vi "Test_Press_Hist.vi"() -> ()   [LabVIEW 2016]
uses:
  <userlib>/Fluigent/Fluigent MFCS/FluigentMFCS_Full.llb/MFCS_EZ Detect.vi
  <userlib>/Fluigent/Fluigent MFCS/FluigentMFCS_Full.llb/MFCS_EZ Initialization.vi
  <userlib>/Fluigent/Fluigent MFCS/FluigentMFCS_Full.llb/MFCS_EZ Read All Channels Pressure.vi
  <vilib>/imath/engines/lvmath2/RunTimeEngine/BuiltInFunctions/sets_unique/NIMS_sets_unique(GV).vi
  <instcachedir>/0/NIMS_sets_unique(GV)_BC60CBD939E647F382369330BF9EA64D.lvgen/NIMS_sets_unique(GV)_BC60CBD939E647F382369330BF9EA64D_001.vi
  <vilib>/imath/engines/lvmath2/RunTimeEngine/BuiltInFunctions/size/NIMS_I32Row=size(GRow).vi
  <instcachedir>/0/NIMS_I32Row=size(GRow)_E5C05C6B13124B29B774CC4F993D3C59.lvgen/NIMS_I32Row=size(GRow)_E5C05C6B13124B29B774CC4F993D3C59_000.vi
  <vilib>/imath/engines/lvmath2/RunTimeEngine/BuiltInFunctions/zeros/NIMS_M=zeros(I32V).vi
  <vilib>/imathl/engines/lvmath/Functions/Error Handling/Create Error.vi
  <vilib>/imath/engines/lvmath2/RunTimeEngine/BuiltInFunctions/length/NIMS_length(GV).vi
  <instcachedir>/0/NIMS_length(GV)_08A3D13377FD4E4B96F5795FBF3698FA.lvgen/NIMS_length(GV)_08A3D13377FD4E4B96F5795FBF3698FA_000.vi
  <vilib>/imath/engines/lvmath2/RunTimeEngine/RangeToken/NIMS_Range_R2 - Integer.vi
  <instcachedir>/0/NIMS_Range_R2 - Integer_416A044C4F024DBE8E97DA138CB3186F.lvgen/NIMS_Range_R2 - Integer_416A044C4F024DBE8E97DA138CB3186F_000.vi
  <vilib>/imath/engines/lvmath2/RunTimeEngine/CommandStatement/MC_CommandStatement_break.vi
  <vilib>/imath/engines/lvmath2/RunTimeEngine/IndexRead/NIMS V(S).vi
  <instcachedir>/0/NIMS V(S)_0488751826AF41519A22953C041130DC.lvgen/NIMS V(S)_0488751826AF41519A22953C041130DC_000.vi
  <vilib>/imath/engines/lvmath2/RunTimeEngine/BuiltInFunctions/findnz/NIMS_[1o]_findnz(GRowV).vi
  <instcachedir>/0/NIMS_[1o]_findnz(GRowV)_656056C849EF4762B1F0843BDDDEF2FF.lvgen/NIMS_[1o]_findnz(GRowV)_656056C849EF4762B1F0843BDDDEF2FF_000.vi
  <instcachedir>/0/NIMS_length(GV)_08A3D13377FD4E4B96F5795FBF3698FA.lvgen/NIMS_length(GV)_08A3D13377FD4E4B96F5795FBF3698FA_002.vi
  <vilib>/imath/engines/lvmath2/RunTimeEngine/IndexReplace/NIMS M(S)=S.vi
  <instcachedir>/0/NIMS M(S)=S_9328EF344EC9443A8B5E4239F1A18A91.lvgen/NIMS M(S)=S_9328EF344EC9443A8B5E4239F1A18A91_000.vi
  <vilib>/imath/engines/lvmath2/RunTimeEngine/ErrorHandling/NIMS_Create Error From Enums.vi
  <vilib>/imath/engines/lvmath2/RunTimeEngine/BuiltInFunctions/difference/NIMS_difference(GV,I32).vi
  <instcachedir>/0/NIMS_difference(GV,I32)_DC7351DCBCF840A8AE147F50EC2CE86E.lvgen/NIMS_difference(GV,I32)_DC7351DCBCF840A8AE147F50EC2CE86E_000.vi
  <vilib>/imath/engines/lvmath2/RunTimeEngine/NodeEndStatement/NIMS_NodeEndStatement_Get Vector.vi
  <instcachedir>/0/NIMS_NodeEndStatement_Get Vector_6D35898B950C4E42AD3C631ACA708625.lvgen/NIMS_NodeEndStatement_Get Vector_6D35898B950C4E42AD3C631ACA708625_000.vi
  <vilib>/imath/engines/lvmath/Functions/Error Handling/MergeErrorsWrapper.vi
  <vilib>/imath/engines/lvmath2/RunTimeEngine/NodeEndStatement/NIMS_NodeEndStatement_Output.vi
  <instcachedir>/0/NIMS_NodeEndStatement_Output_53EC0D466D134D7ABD903AC30B43404B.lvgen/NIMS_NodeEndStatement_Output_53EC0D466D134D7ABD903AC30B43404B_005.vi
  <instcachedir>/0/NIMS_NodeEndStatement_Output_53EC0D466D134D7ABD903AC30B43404B.lvgen/NIMS_NodeEndStatement_Output_53EC0D466D134D7ABD903AC30B43404B_004.vi
  <vilib>/imath/engines/lvmath2/RunTimeEngine/ErrorHandling/NIMS_Finalize Error.vi
  <userlib>/Fluigent/Fluigent MFCS/FluigentMFCS_Full.llb/MFCS_EZ Write Channel Pressure.vi
  <vilib>/Analysis/NI_AALPro.lvlib
panel:
  out "diffz":dbl[](array[numeric])
  out "num":i32[](array[numeric])
  out "unique_nums":dbl[](array[numeric])
  in  "Reset Bins":bool
  in  "stop":bool
  out "Histogram Graph 2":T1(graph)
  out "Histogram Graph":T1(graph)
  in  "Pressure Channels":i16[](array[numeric])=[2, 3]
  in  "Manual Pressure Set":dbl[](array[numeric])=[400.0, 400.0] format="%_7g"
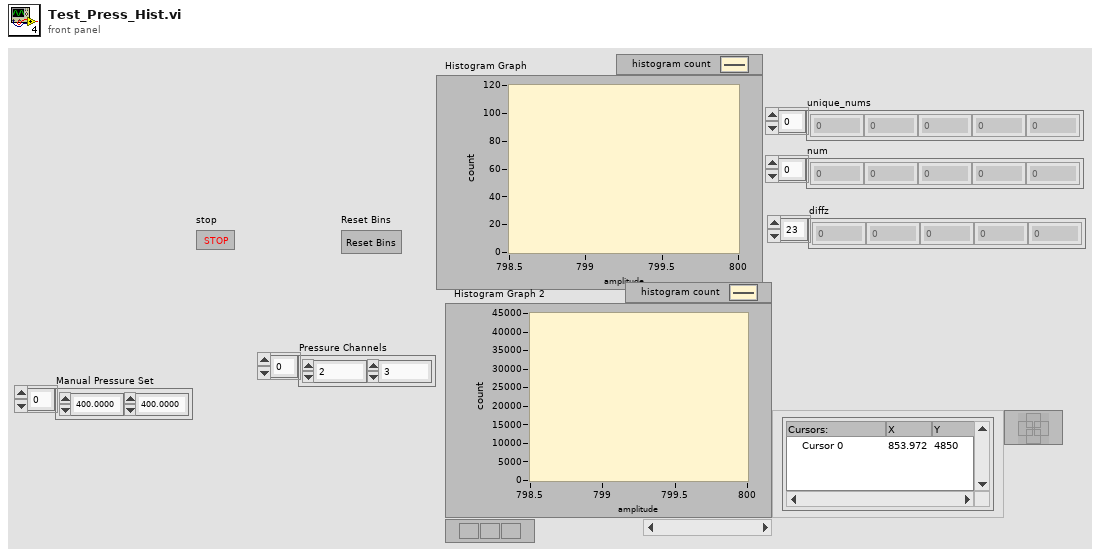
[diagram p1: front panel]
types:
  T1 = cluster{"X Values":dbl[], "Histogram: h(x)":i32[]}
  T2 = typedef "_EZmfcsSN.ctl" = u16
  T3 = typedef "_EZmfcsRefNum.ctl" = refnum<k1>
  T4 = cluster{"lower":dbl, "upper":dbl, "inclusion":u32}[]
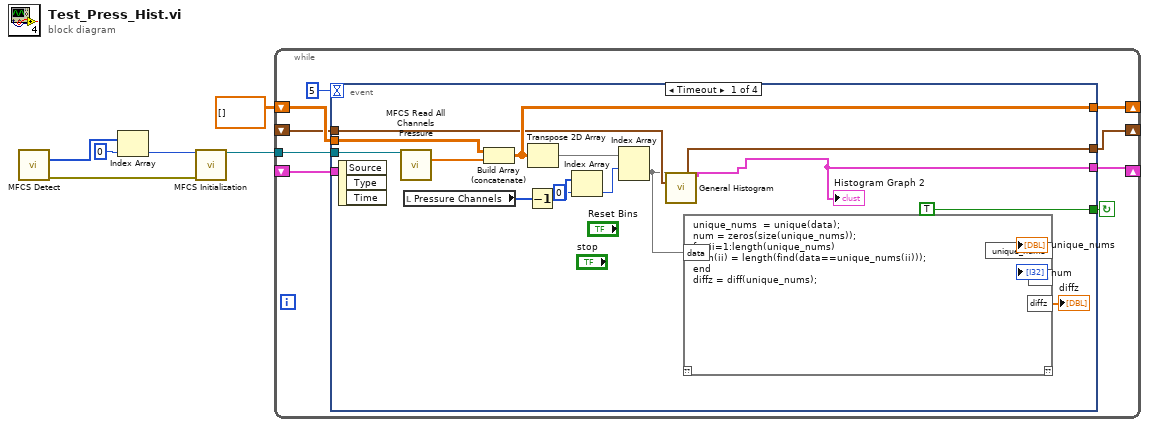
[diagram p0: block diagram]
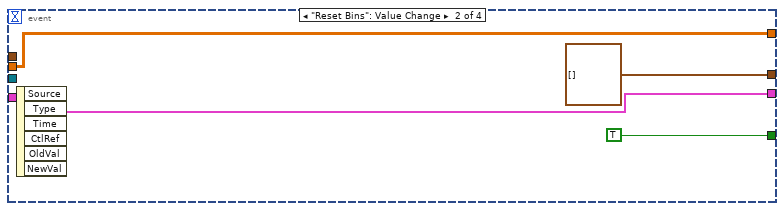
[diagram p2: hidden frame]
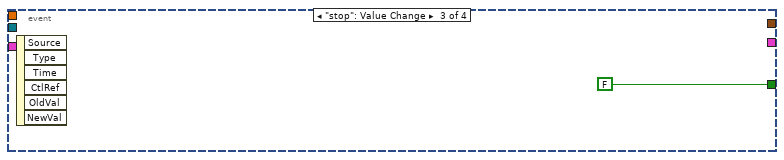
[diagram p3: hidden frame]
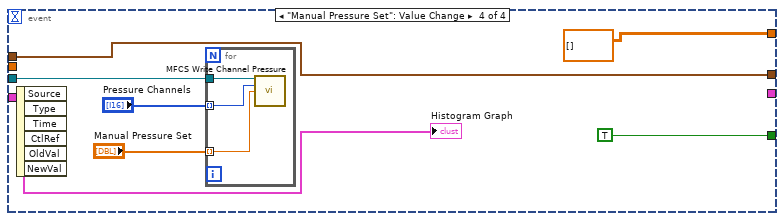
[diagram p4: hidden frame]
diagram:
  n1 = call-poly <userlib>:"MFCS Detect.vi"() -> ("[SN MFCS_EZ]"=w6:T2[], "error out"=w4:errorcluster)  [unwired: 14 in]
  n2 = Index Array(array=w6, index=0) -> (element=w5:T2)
  n3 = call-poly <userlib>:"MFCS Initialization.vi"("SN MFCS_EZ"=w5, "error in (no error)"=w4) -> ("MFCS_EZ"=w2:T3)  [unwired: 11 in, 2 out]
  n4 = while {
    tunnel: w2 -> [w15]
    shift-right: [w11] -> _
    shift-left: dbl[][] [] -> [w12]
    shift-right: [w10] -> _
    shift-left: _ -> [w9]
    shift-right: [w8] -> _
    shift-left: _ -> [w7]
    stop <- w13 continue-if-true
    n5 = event shown="[0] Timeout" {
      selector: _ -> [_ _ _ _]
      dyn-events: _ -> [_ _ _ _]
      timeout: 5 -> [_ _ _ _]
      tunnel: w15 -> [w32 _ _ w156]
      tunnel: [TRUE TRUE FALSE TRUE] -> w13
      tunnel: w12 -> [w29 w151 _ _]
      tunnel: [w28 w151 _ dbl[][] []] -> w11
      tunnel: [w22 w150 _ _] -> w10
      tunnel: w9 -> [_ w150 _ w155]
      tunnel: [w21 T4 [] ("Bins Out") _ w154] -> w8
      tunnel: w7 -> [w20 _ _ w154]
      event Timeout {
        n6 = event-data() -> ()  [unwired: 1 in, 3 out]
        n7 = call-poly <userlib>:"MFCS Read All Channels Pressure.vi"("MFCS_EZ"=w32) -> ("All Channels Pressure"=w30:dbl[])  [unwired: 12 in, 2 out]
        n8 = local read "Pressure Channels"() -> (w31:i16[])
        n9 = Build Array (concatenate)(w29, w30) -> (w28:dbl[][])
        n10 = Decrement(x=w31) -> (x-1=w25:i16[])
        n11 = Transpose 2D Array(2D array=w28) -> (transposed array=w26:dbl[][])
        n12 = Index Array(array=w25, index=0) -> (element=w23:i16)
        n13 = Index Array(array=w26, index (row)=w23) -> (element=w19:dbl[])  [unwired: 1 in]
        n14 = call <vilib>:"General Histogram.vi"("X"=w19, "Bins"=w20) -> ("Bins Out"=w21:T4, "Histogram Graph"=w22:T1)  [unwired: 8 in, 4 out]
        "Histogram Graph 2" <- w22
        n15 = mathscript code="unique_nums  = unique(data);\nnum = zeros(size(unique_nums));\nfor ii=1:length(unique_nums)\nnum(ii) = length(find(data==unique_nums(ii)));\nend\ndiffz = diff(unique_nums);"("data"=w19) -> ("num"=→"num":i32[], "unique_nums"=→"unique_nums":dbl[], "diffz"=→"diffz":dbl[])  [unwired: 1 in, 1 out]
      }
      event "Reset Bins": Value Change {
        n16 = event-data() -> ()  [unwired: 1 in, 6 out]
      }
      event "stop": Value Change {
        n17 = event-data() -> ()  [unwired: 1 in, 6 out]
      }
      event "Manual Pressure Set": Value Change {
        n18 = event-data() -> ()  [unwired: 1 in, 6 out]
        n19 = for {
          tunnel: "Manual Pressure Set" -> [w163] mode=indexing
          tunnel: "Pressure Channels" -> [w162] mode=indexing
          tunnel: w156 -> [w161]
          n20 = call-poly <userlib>:"MFCS Write Channel Pressure.vi"("MFCS_EZ"=w161, "Channel Number (default=1)"=w162, "Pressure (mBar)"=w163) -> ()  [unwired: 11 in, 2 out]
        }
        "Histogram Graph" <- w155
      }
    }
  }
